vi "Sync Tasks-PXIe-433x.vi"(8 "error in":errorcluster, 11 "Task(s) in":refnum<k21>[](array[refnum])) -> (0 "error out":errorcluster, 3 "Task(s) out":refnum<k21>[](array[refnum]))   [LabVIEW 2022 SP3]
doc: "This subVI synchronizes multiple tasks of 433x devices together. It shares a SyncPulse, sets the SyncClock Interval, Reset Delay, and MinDelayToStart of each task appropriately."
uses:
  <vilib>/gmath/NI_Gmath.lvlib
  <resource>/objmgr/daqmx.rc
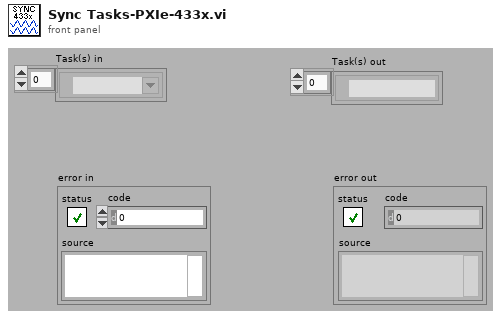
[diagram p1: front panel]
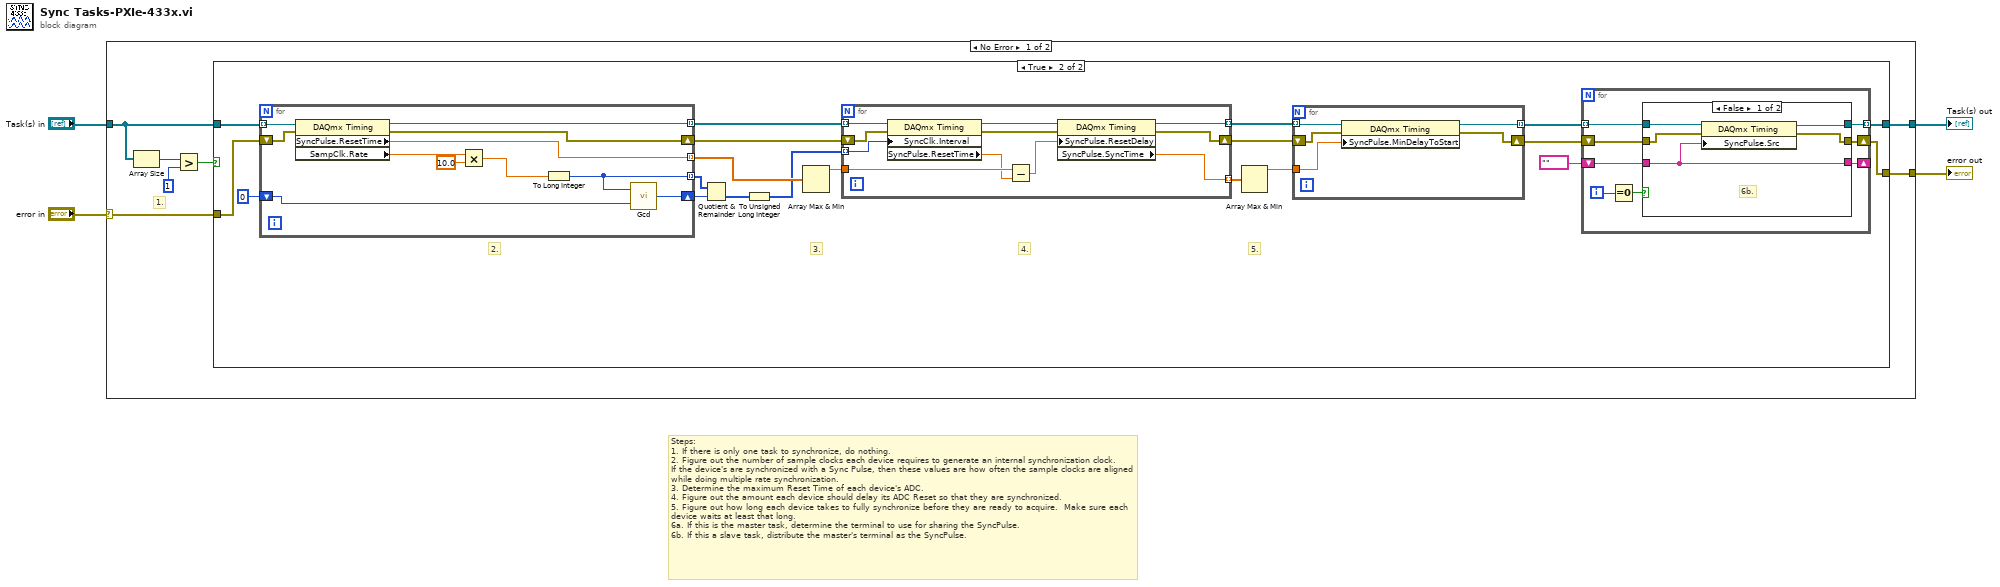
[diagram p0: block diagram]
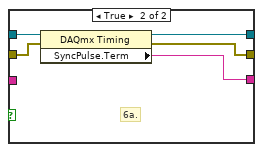
[diagram p3: hidden frame]
diagram:
  # "Steps:\n1. If there is only one task to synchronize, do nothing.\n2. Figure out the number of sample clocks each device requires to generate an internal synchronization clock.  \nIf the device's are synchronized with a Sync Pulse, then these values are how often the sample clocks are aligned \nwhile doing multiple rate synchronization.\n3. Determine the maximum Reset Time of each device's ADC.\n4. Figure out the amount each device should delay its ADC Reset so that they are synchronized.\n5. Figure out how long each device takes to fully synchronize before they are ready to acquire.  Make sure each \ndevice waits at least that long.\n6a. If this is the master task, determine the terminal to use for sharing the SyncPulse.\n6b. If this a slave task, distribute the master's terminal as the SyncPulse."
  n1 = case shown="No Error" "error in" {
    selector: "error in" -> [w5 w80]
    tunnel: [w6 w80] -> w3
    tunnel: [w7 w79] -> w2
    tunnel: "Task(s) in" -> [w8 w79]
    frame No Error {
      # "1."
      n2 = Array Size(array=w8) -> (size(s)=w11:i32)
      n3 = Greater?(x=w11, y=1) -> (0:w9:bool)
      n4 = case shown="True" w9 {
        tunnel: w8 -> [w13 w27]
        tunnel: [w13 w20] -> w7
        tunnel: [w12 w21] -> w6
        tunnel: w5 -> [w12 w26]
        frame False {
        }
        frame True {
          # "5."
          # "4."
          # "3."
          # "2."
          n5 = for {
            tunnel: w27 -> [w78] mode=indexing
            shift-right: [w76] -> w25
            shift-left: w26 -> [w77]
            tunnel: [w75] -> w33 mode=indexing
            tunnel: [w73] -> w19 mode=indexing
            shift-right: [w70] -> w14
            shift-left: 0 ("lcm(x,y)") -> [w71]
            tunnel: [w72] -> w15 mode=indexing
            n6 = property class="DAQmx Timing"(reference=w78, error in=w77) -> (reference out=w75:refnum<k21>, error out=w76:errorcluster, "SyncPulse.ResetTime"=w73:dbl, "SampClk.Rate"=w74:dbl)
            n7 = Multiply(x=w74, y=10.0) -> (x*y=w68:dbl)
            n8 = To Long Integer(number=w68) -> (32bit integer=w72:i32)
            n9 = call <vilib>:"Gcd.vi"("y"=w71, "x"=w72) -> ("gcd(x,y)"=w70:i32)
          }
          n10 = Quotient & Remainder(x=w15, y=w14) -> (floor(x/y)=w17:i32[])  [unwired: 1 out]
          n11 = To Unsigned Long Integer(number=w17) -> (unsigned 32bit integer=w16:u32[])
          n12 = Array Max & Min(array=w19) -> (max value=w32:dbl)  [unwired: 3 out]
          n13 = for {
            shift-right: [w61] -> w29
            shift-left: w25 -> [w67]
            tunnel: w33 -> [w66] mode=indexing
            tunnel: w32 -> [w63]
            tunnel: [w60] -> w30 mode=indexing
            tunnel: [w59] -> w31 mode=indexing
            tunnel: w16 -> [w57] mode=indexing
            n14 = property class="DAQmx Timing"(reference=w66, error in=w67, "SyncClk.Interval"=w57) -> (reference out=w65:refnum<k21>, error out=w64:errorcluster, "SyncPulse.ResetTime"=w58:dbl)
            n15 = Subtract(x=w63, y=w58) -> (x-y=w62:dbl)
            n16 = property class="DAQmx Timing"(reference=w65, error in=w64, "SyncPulse.ResetDelay"=w62) -> (reference out=w60:refnum<k21>, error out=w61:errorcluster, "SyncPulse.SyncTime"=w59:dbl)
          }
          n17 = Array Max & Min(array=w31) -> (max value=w28:dbl)  [unwired: 3 out]
          n18 = for {
            shift-right: [w55] -> w22
            shift-left: w29 -> [w56]
            tunnel: [w54] -> w23 mode=indexing
            tunnel: w30 -> [w53] mode=indexing
            tunnel: w28 -> [w52]
            n19 = property class="DAQmx Timing"(reference=w53, error in=w56, "SyncPulse.MinDelayToStart"=w52) -> (reference out=w54:refnum<k21>, error out=w55:errorcluster)
          }
          n20 = for {
            tunnel: w23 -> [w39] mode=indexing
            tunnel: [w38] -> w20 mode=indexing
            shift-right: [w37] -> _
            shift-left: tag "" ("SyncPulse.Term") -> [w34]
            shift-right: [w35] -> w21
            shift-left: w22 -> [w36]
            i -> [w41]
            n21 = Equal To 0?(x=w41) -> (x = 0?=w40:bool)
            n22 = case shown="False" w40 {
              tunnel: w39 -> [w46 w51]
              tunnel: [w44 w50] -> w38
              tunnel: [w43 w49] -> w37
              tunnel: w36 -> [w42 w48]
              tunnel: [w45 w47] -> w35
              tunnel: w34 -> [w43 _]
              frame False {
                # "6b."
                n23 = property class="DAQmx Timing"(reference=w46, error in=w42, "SyncPulse.Src"=w43) -> (reference out=w44:refnum<k21>, error out=w45:errorcluster)
              }
              frame True {
                # "6a."
                n24 = property class="DAQmx Timing"(reference=w51, error in=w48) -> (reference out=w50:refnum<k21>, error out=w47:errorcluster, "SyncPulse.Term"=w49:tag)
              }
            }
          }
        }
      }
    }
    frame Error {
    }
  }
  "Task(s) out" <- w2
  "error out" <- w3
